vi "ambient_air_pressure_correction.vi"(11 "Numeric in":dbl) -> (3 "Numeric out":dbl)   [LabVIEW 2014]
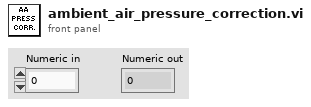
[diagram p1: front panel]
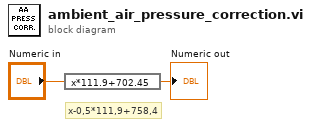
[diagram p0: block diagram]
diagram:
  # "x-0,5*111,9+758,4"
  n1 = expression code="x*111.9+702.45"("Numeric in") -> (→"Numeric out":dbl)
